vi "Stop Task Wrapper.vi"(0 "Task map in":map{string, refnum<k21>}(c390), 5 "Message Data in":T2, 11 "error in (no error)":errorcluster) -> (4 "Task map out":map{string, refnum<k21>}(c390), 6 "Message Data out":T1, 15 "error out":errorcluster)   [LabVIEW 2021, in "NI DAQmx_wrapper.lvlib"]
uses:
  NI DAQmx_wrapper.lvlib
  NI DAQmx_server/RPC Messages/nidaqmx_grpc_StopTaskRequest.ctl
  NI DAQmx_server/RPC Messages/nidevice_grpc_Session_session/nidevice_grpc_Session_session.lvclass
  NI DAQmx_server/RPC Messages/nidevice_grpc_Session.ctl
  NI DAQmx_server/RPC Messages/nidaqmx_grpc_StopTaskResponse.ctl
  NI DAQmx_server/RPC Messages/nidevice_grpc_Session_session/nidevice_grpc_Session_session.lvclass/nidevice_grpc_Session_session.ctl
  NI DAQmx_server/NI DAQmx_server.lvlib
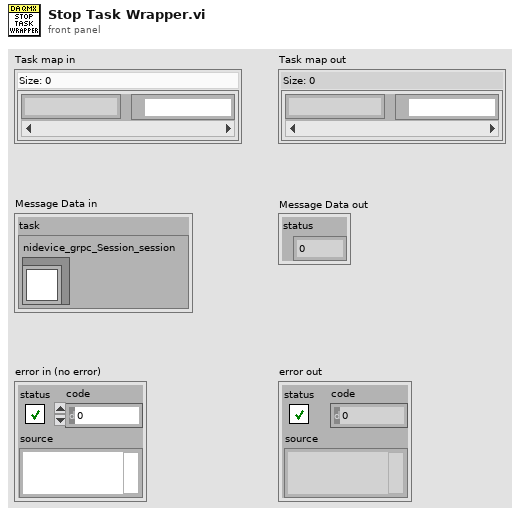
[diagram p1: front panel]
types:
  T1 = typedef "NI DAQmx_server.lvlib/nidaqmx_grpc_StopTaskResponse.ctl" = cluster{"status":i32}
  T2 = typedef "NI DAQmx_server.lvlib/nidaqmx_grpc_StopTaskRequest.ctl" = cluster{"task":T3}
  T3 = typedef "NI DAQmx_server.lvlib/nidevice_grpc_Session.ctl" = cluster{"nidevice_grpc_Session_session":refnum<class "nidevice_grpc_Session_session.lvclass">}
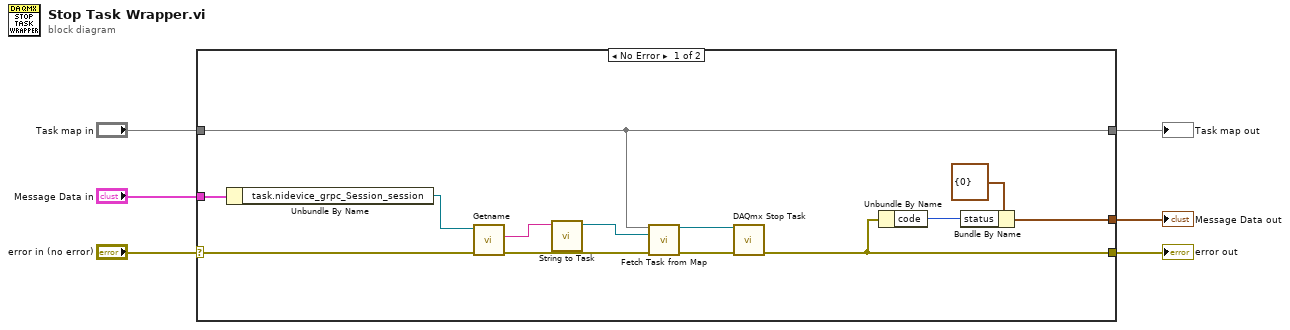
[diagram p0: block diagram]
diagram:
  n1 = case shown="No Error" "error in (no error)" {
    selector: "error in (no error)" -> [w15 w21]
    tunnel: [w9 w21] -> w5
    tunnel: "Task map in" -> [w13 w20]
    tunnel: [w13 w20] -> w3
    tunnel: "Message Data in" -> [w19 _]
    tunnel: [w7 _] -> w1
    frame No Error {
      n2 = Unbundle By Name(w19) -> ("task.nidevice_grpc_Session_session"=w14:refnum<class "nidevice_grpc_Session_session.lvclass">)
      n3 = call "Getname.vi"("error in (no error)"=w15, "OneOfTemplate in"=w14) -> ("error out"=w18:errorcluster, "Get_Val"=w17:string)  [unwired: 7 in, 1 out]
      n4 = call "String to Task.vi"("Get_Val"=w17) -> ("Refnum out"=w16:refnum<k21>)  [unwired: 10 in]
      n5 = call "Fetch Task from Map.vi"("Task map in"=w13, "Task in"=w16, "error in (no error)"=w18) -> ("Task out"=w11:refnum<k21>, "error out"=w12:errorcluster)  [unwired: 10 in, 1 out]
      n6 = call <vilib>:"DAQmx Stop Task.vi"("task/channels in"=w11, "error in"=w12) -> ("error out"=w9:errorcluster)  [unwired: 12 in, 1 out]
      n7 = Unbundle By Name(w9) -> ("code"=w10:i32)
      n8 = Bundle By Name(cluster=T1 {"status"=0} ("Message Data 2"), "status"=w10) -> (w7:T1)
    }
    frame Error {
    }
  }
  "error out" <- w5
  "Task map out" <- w3
  "Message Data out" <- w1
